vi "libtiff3_write_tiff page 16bit.vi"(0 "Handle":i32, 1 "Image Pixels (U16)":u16[][](array[numeric]), 4 "ImageDescription":string, 5 "error in (no error)":errorcluster, 6 "page":u32, 7 "x.pixels":i32, 8 "totalpages":i32, 9 "y.pixels":i32) -> (14 "Handle out":i32, 19 "error out":errorcluster)   [LabVIEW 2012]
doc: "SciScan 1.2 160622\nWrite a SGL (32-bit IEEE) page using LIBTIFFwriteScanLine to a file previously open for writing"
uses:
  Libtiff3/libtiff3.dll
panel:
  out "status_compression":i32
  out "status width":i32
  out "status_length":i32
  out "status_spp":i32
  out "status_bps":i32
  out "status_orientation":i32
  out "status_planarconfig":i32
  out "status_photo":i32
  out "status_writscanline":i32
  out "status_subfile":i32
  out "status_writedir":i32
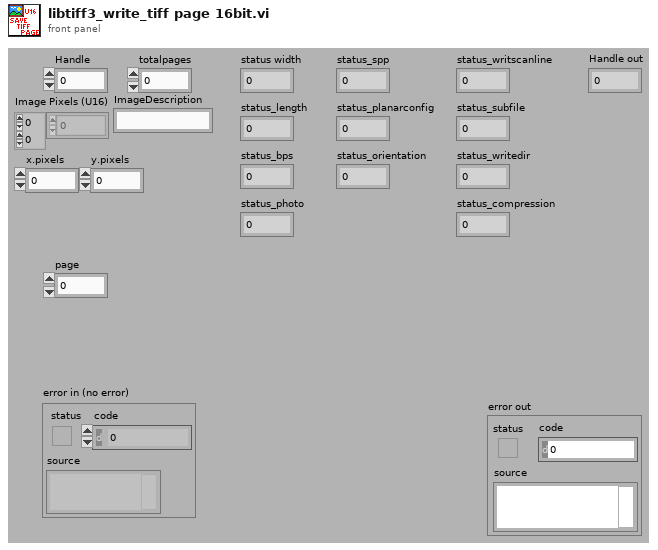
[diagram p1: front panel]
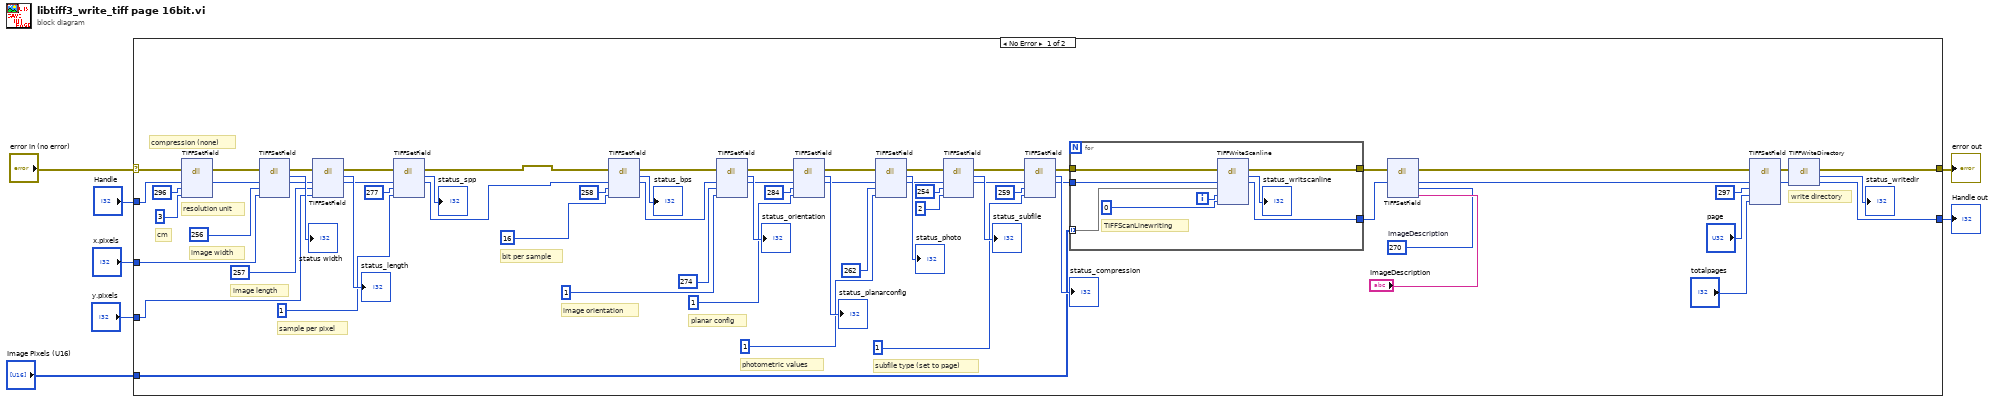
[diagram p0: block diagram]
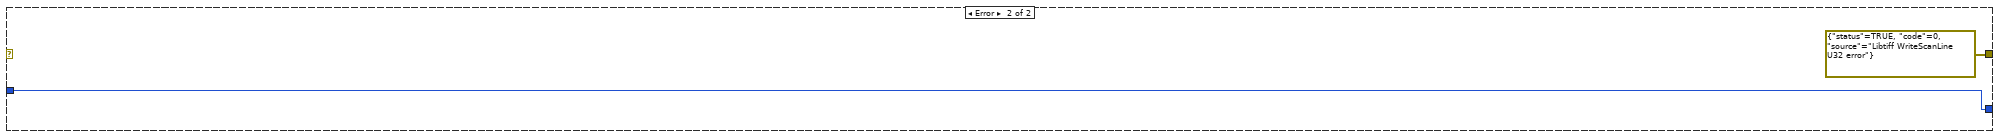
[diagram p2: hidden frame]
diagram:
  n1 = case shown="No Error" "error in (no error)" {
    selector: "error in (no error)" -> [w20 _]
    tunnel: "Handle" -> [w21 w83]
    tunnel: [w45 w83] -> w1
    tunnel: [w33 errorcluster {"status"=TRUE, "code"=0, "source"="Libtiff WriteScanLine U32 error"} ("error out")] -> w6
    tunnel: "Image Pixels (U16)" -> [w26 _]
    tunnel: "x.pixels" -> [w25 _]
    tunnel: "y.pixels" -> [w24 _]
    frame No Error {
      w12 = 270  # ImageDescription
      # "cm"
      # "resolution unit"
      # "compression (none)"
      # "write directory"
      # "subfile type (set to page)"
      # "photometric values"
      # "planar config"
      # "image orientation"
      # "bit per sample"
      # "sample per pixel"
      # "image length"
      # "image width"
      n2 = dll-call lib="D:/gitrepo/140812_ssdev_repo/Libtiff3/libtiff3.dll" fn="TIFFSetField"(error in=w20, "Handle"=w21, "TIFF_tag"=296, "value"=u32 3) -> (error out=w19:errorcluster, "Handle"=w18:i32)  [unwired: 4 in, 2 out]
      n3 = dll-call lib="D:/gitrepo/140812_ssdev_repo/Libtiff3/libtiff3.dll" fn="TIFFSetField"(error in=w19, "Handle"=w18, "TIFF_tag"=256, "Value"=w25) -> (error out=w40:errorcluster, "return type"=→"status width":i32, "Handle"=w71:i32)  [unwired: 4 in, 1 out]
      n4 = dll-call lib="D:/gitrepo/140812_ssdev_repo/Libtiff3/libtiff3.dll" fn="TIFFSetField"(error in=w40, "Handle"=w71, "TIFF_tag"=257, "value"=w24) -> (error out=w39:errorcluster, "return type"=→"status_length":i32, "Handle"=w68:i32)  [unwired: 4 in, 1 out]
      n5 = dll-call lib="D:/gitrepo/140812_ssdev_repo/Libtiff3/libtiff3.dll" fn="TIFFSetField"(error in=w39, "Handle"=w68, "TIFF_tag"=277, "value"=u32 1) -> (error out=w9:errorcluster, "return type"=→"status_spp":i32, "Handle"=w8:i32)  [unwired: 4 in, 1 out]
      n6 = dll-call lib="D:/gitrepo/140812_ssdev_repo/Libtiff3/libtiff3.dll" fn="TIFFSetField"(error in=w9, "Handle"=w8, "TIFF_tag"=258, "value"=u32 16) -> (error out=w38:errorcluster, "return type"=→"status_bps":i32, "Handle"=w63:i32)  [unwired: 4 in, 1 out]
      n7 = dll-call lib="D:/gitrepo/140812_ssdev_repo/Libtiff3/libtiff3.dll" fn="TIFFSetField"(error in=w38, "Handle"=w63, "TIFF_tag"=274, "value"=u32 1) -> (error out=w37:errorcluster, "return type"=→"status_orientation":i32, "Handle"=w59:i32)  [unwired: 4 in, 1 out]
      n8 = dll-call lib="D:/gitrepo/140812_ssdev_repo/Libtiff3/libtiff3.dll" fn="TIFFSetField"(error in=w37, "Handle"=w59, "TIFF_tag"=284, "value"=u32 1) -> (error out=w36:errorcluster, "return type"=→"status_planarconfig":i32, "Handle"=w55:i32)  [unwired: 4 in, 1 out]
      n9 = dll-call lib="D:/gitrepo/140812_ssdev_repo/Libtiff3/libtiff3.dll" fn="TIFFSetField"(error in=w36, "Handle"=w55, "TIFF_tag"=262, "value"=u32 1) -> (error out=w35:errorcluster, "return type"=→"status_photo":i32, "Handle"=w50:i32)  [unwired: 4 in, 1 out]
      n10 = dll-call lib="D:/gitrepo/140812_ssdev_repo/Libtiff3/libtiff3.dll" fn="TIFFSetField"(error in=w35, "Handle"=w50, "TIFF_tag"=254, "value"=u32 2) -> (error out=w34:errorcluster, "return type"=→"status_subfile":i32, "Handle"=w42:i32)  [unwired: 4 in, 1 out]
      n11 = dll-call lib="D:/gitrepo/140812_ssdev_repo/Libtiff3/libtiff3.dll" fn="TIFFSetField"(error in=w34, "Handle"=w42, "TIFF_tag"=259, "value"=u32 1) -> (error out=w17:errorcluster, "return type"=→"status_compression":i32, "Handle"=w16:i32)  [unwired: 4 in, 1 out]
      n12 = for {
        tunnel: [w74] -> w10
        tunnel: [w76] -> w11
        tunnel: w16 -> [w80]
        tunnel: w17 -> [w81]
        tunnel: w26 -> [w79] mode=indexing
        i -> [w78]
        # "TIFFScanLinewriting"
        n13 = dll-call lib="D:/gitrepo/140812_ssdev_repo/Libtiff3/libtiff3.dll" fn="TIFFWriteScanline"(error in=w81, "Handle"=w80, "buffer"=w79, "row"=w78, "sample"=0) -> (error out=w76:errorcluster, "return type"=→"status_writscanline":i32, "Handle"=w74:i32)  [unwired: 5 in, 1 out]
      }
      n14 = dll-call lib="D:/gitrepo/140812_ssdev_repo/Libtiff3/libtiff3.dll" fn="TIFFSetField"(error in=w11, "Handle"=w10, "TIFF_tag"=w12, "Value"="ImageDescription") -> (error out=w15:errorcluster, "Handle"=w14:i32)  [unwired: 4 in, 2 out]
      n15 = dll-call lib="D:/gitrepo/140812_ssdev_repo/Libtiff3/libtiff3.dll" fn="TIFFSetField"(error in=w15, "Handle"=w14, "TIFF_tag"=297, "page"="page", "totalpages"="totalpages") -> (error out=w28:errorcluster, "Handle"=w27:i32)  [unwired: 5 in, 2 out]
      n16 = dll-call lib="D:/gitrepo/140812_ssdev_repo/Libtiff3/libtiff3.dll" fn="TIFFWriteDirectory"(error in=w28, "Handle"=w27) -> (error out=w33:errorcluster, "return type"=→"status_writedir":i32, "Handle"=w45:i32)  [unwired: 2 in, 1 out]
    }
    frame Error {
    }
  }
  "Handle out" <- w1
  "error out" <- w6
